vi "AddVirtual.vi"(8 "error in (no error)":errorcluster, 10 "AllVirtualTypeData":T1={"Search Name"="", "Start X"=0.0, "Increase X"=0.0, "X Step"=1, "Start Y"=0.0, "Increase Y"=0.0, "Y Step"=1, "Sensor"=0} {"Y Step" min=1 step=1; "X Step" min=1 step=1}, 11 "Project.lvclass In":refnum<class "Project.lvclass">) -> (0 "error out":errorcluster, 3 "Project.lvclass Out":refnum<class "Project.lvclass">)   [LabVIEW 2014, in "Project.lvclass"]
uses:
  Project.lvclass
  Virtual/Control/AllVirtualTypeData.ctl
  VirtualSetupDataTypeDefine.ctl
  Project.lvclass/Project.ctl
  Virtual/VirtualOrigin.lvclass
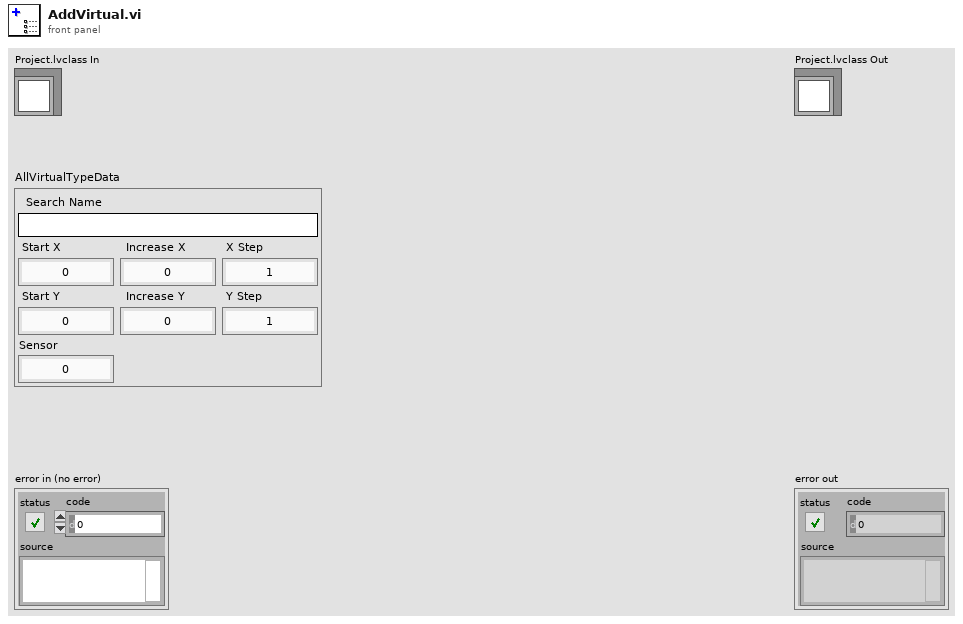
[diagram p1: front panel]
types:
  T1 = typedef "VirtualOrigin.lvclass/AllVirtualTypeData.ctl" = cluster{"Search Name":string, "Start X":dbl, "Increase X":dbl, "X Step":i32, "Start Y":dbl, "Increase Y":dbl, "Y Step":i32, "Sensor":i32}
  T2 = typedef "Project.lvclass/VirtualSetupDataTypeDefine.ctl" = T1[]
  T3 = typedef "Project.lvclass/ProjectDataTableTypeDefine.ctl" = string[][]
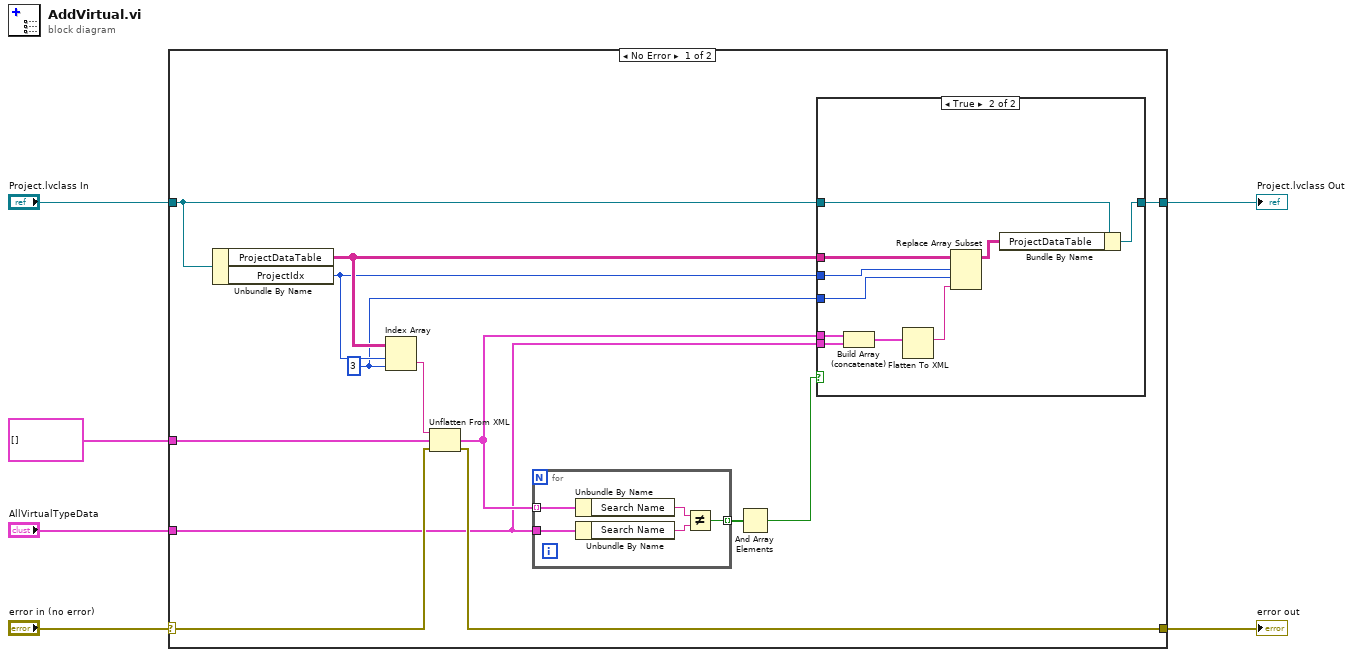
[diagram p0: block diagram]
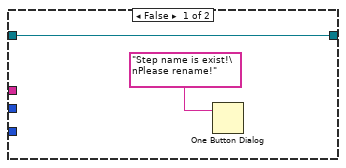
[diagram p2: hidden frame]
diagram:
  n1 = case shown="No Error" "error in (no error)" {
    selector: "error in (no error)" -> [w13 w38]
    tunnel: [w10 w38] -> w5
    tunnel: "Project.lvclass In" -> [w16 w37]
    tunnel: [w15 w37] -> w3
    tunnel: T2 [] ("VirtualSetupClusterArray") -> [w8 _]
    tunnel: "AllVirtualTypeData" -> [w7 _]
    frame No Error {
      w17 = 3 ("disabled index (col)")
      n2 = Unbundle By Name(w16) -> ("ProjectDataTable"=w19:T3, "ProjectIdx"=w18:i32)
      n3 = Index Array(array=w19, index (row)=w18, index (col)=w17) -> (element=w14:string)
      n4 = Unflatten From XML(xml string=w14, type=w8, error in (no error)=w13) -> (value=w9:T2, error out=w10:errorcluster)
      n5 = for {
        tunnel: w9 -> [w24] mode=indexing
        tunnel: [w22] -> w12 mode=indexing
        tunnel: w7 -> [w21]
        n6 = Unbundle By Name(w24) -> ("Search Name"=w23:string)
        n7 = Unbundle By Name(w21) -> ("Search Name"=w20:string)
        n8 = Not Equal?(x=w23, y=w20) -> (x != y?=w22:bool)
      }
      n9 = And Array Elements(Boolean array=w12) -> (logical AND=w11:bool)
      n10 = case shown="True" w11 {
        tunnel: w19 -> [_ w36]
        tunnel: w18 -> [_ w35]
        tunnel: w17 -> [_ w34]
        tunnel: w16 -> [w26 w33]
        tunnel: [w26 w31] -> w15
        tunnel: w9 -> [_ w29]
        tunnel: w7 -> [_ w28]
        frame False {
          n11 = One Button Dialog(message="Step name is exist!\nPlease rename!") -> ()  [unwired: 1 in, 1 out]
        }
        frame True {
          n12 = Build Array (concatenate)(w29, w28) -> (w30:T2)
          n13 = Flatten To XML(anything=w30) -> (xml string=w27:string)
          n14 = Replace Array Subset(array=w36, new element=w27, index (row)=w35, index (col)=w34) -> (w32:T3)
          n15 = Bundle By Name(cluster=w33, "ProjectDataTable"=w32) -> (w31:refnum<class "Project.lvclass">)
        }
      }
    }
    frame Error {
    }
  }
  "error out" <- w5
  "Project.lvclass Out" <- w3
